vi "Acquisition simulator.vi"() -> ()   [LabVIEW 2017]
uses:
  Rendezvous global.vi
panel:
  out "End":bool
  out "Running":bool
  out "Rendezvous":bool
  out "Initial config":bool
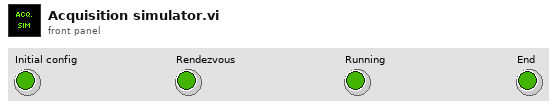
[diagram p1: front panel]
types:
  T1 = typedef "Rendezvous RefNum" = refnum<k1>
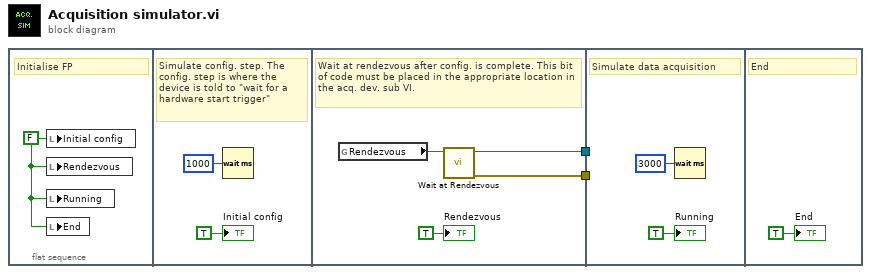
[diagram p0: block diagram]
diagram:
  n1 = flat-sequence {
    tunnel: [w8] -> w2
    tunnel: [w7] -> w1
    tunnel: w2 -> [_]
    tunnel: w1 -> [_]
    frame #0 {
      w3 = FALSE ("Initial config")
      # "Initialise FP"
      n2 = local write "Initial config"(w3) -> ()
      n3 = local write "Rendezvous"(w3) -> ()
      n4 = local write "Running"(w3) -> ()
      n5 = local write "End"(w3) -> ()
    }
    frame #1 {
      # "Simulate config. step. The config. step is where the device is told to \"wait for a hardware start trigger\""
      n6 = Wait (ms)(milliseconds to wait=u32 1000) -> ()  [unwired: 1 out]
      "Initial config" <- TRUE ("Initial config")
    }
    frame #2 {
      # "Wait at rendezvous after config. is complete. This bit of code must be placed in the appropriate location in the acq. dev. sub VI."
      n7 = global read "Rendezvous global.vi" "Rendezvous"() -> (w6:T1)
      n8 = call <vilib>:"Wait at Rendezvous.vi"("rendezvous"=w6) -> ("error out"=w7:errorcluster, "rendezvous out"=w8:T1)  [unwired: 4 in, 1 out]
      "Rendezvous" <- TRUE ("Initial config")
    }
    frame #3 {
      # "Simulate data acquisition"
      n9 = Wait (ms)(milliseconds to wait=u32 3000) -> ()  [unwired: 1 out]
      "Running" <- TRUE ("Initial config")
    }
    frame #4 {
      # "End"
      "End" <- TRUE ("Initial config")
    }
  }
